vi "iRobot Sensor Stream Process (all sensors).vi"(11 "stream in":u8[](array[numeric])) -> (1 "sensors":T1 {"Infrared" format="%02x"}, 2 "Packet Found?":bool, 3 "stream out":u8[](array[numeric]))   [LabVIEW 2010]
doc: "Process a stream of UART communication and extract a sensor packet.\n\nFor simplicity, this VI assumes that the robot is streaming Sensor Group 6, which contains all sensor data."
uses:
  Sensor Controls/iRobot Sensor Group 6.ctl
  Sensor Controls/iRobot Bumps + Wheel Drops.ctl
  Sensor Controls/iRobot Low-Side Driver + Wheel Overcurrent.ctl
  Sensor Controls/iRobot Buttons.ctl
  Sensor Controls/iRobot Charging State.ctl
  Sensor Controls/iRobot Cargo Bay Digital Inputs.ctl
  Sensor Controls/iRobot Charging Sources Available.ctl
  Sensor Controls/iRobot OI Mode.ctl
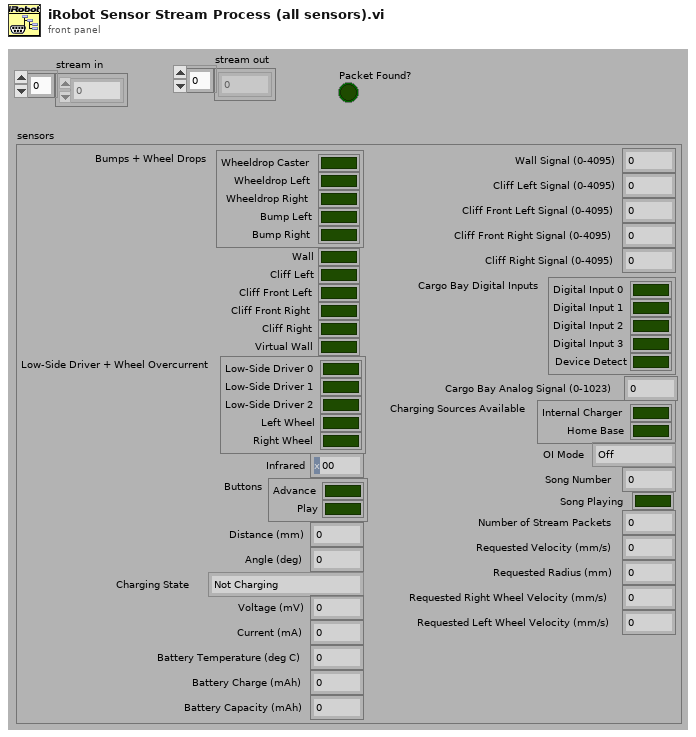
[diagram p1: front panel]
types:
  T1 = typedef "iRobot Sensor Group 6.ctl" = cluster{"Bumps + Wheel Drops":T2, "Wall":bool, "Cliff Left":bool, "Cliff Front Left":bool, "Cliff Front Right":bool, "Cliff Right":bool, "Virtual Wall":bool, "Low-Side Driver + Wheel Overcurrent":T3, "Infrared":u8, "Buttons":T4, "Distance (mm)":i32, "Angle (deg)":i32, "Charging State":T5, "Voltage (mV)":u16, "Current (mA)":i16, "Battery Temperature (deg C)":i8, "Battery Charge (mAh)":u16, "Battery Capacity (mAh)":u16, "Wall Signal (0-4095)":u16, "Cliff Left Signal (0-4095)":u16, "Cliff Front Left Signal (0-4095)":u16, "Cliff Front Right Signal (0-4095)":u16, "Cliff Right Signal (0-4095)":u16, "Cargo Bay Digital Inputs":T6, "Cargo Bay Analog Signal (0-1023)":u16, "Charging Sources Available":T7, "OI Mode":T8, "Song Number":u8, "Song Playing":bool, "Number of Stream Packets":u8, "Requested Velocity (mm/s)":u8, "Requested Radius (mm)":u8, "Requested Right Wheel Velocity (mm/s)":u8, "Requested Left Wheel Velocity (mm/s)":u8}
  T2 = typedef "iRobot Bumps + Wheel Drops.ctl" = cluster{"Wheeldrop Caster":bool, "Wheeldrop Left":bool, "Wheeldrop Right":bool, "Bump Left":bool, "Bump Right":bool}
  T3 = typedef "iRobot Low-Side Driver + Wheel Overcurrent.ctl" = cluster{"Low-Side Driver 0":bool, "Low-Side Driver 1":bool, "Low-Side Driver 2":bool, "Left Wheel":bool, "Right Wheel":bool}
  T4 = typedef "iRobot Buttons.ctl" = cluster{"Advance":bool, "Play":bool}
  T5 = typedef "iRobot Charging State.ctl" = enum16{"Not Charging", "Reconditioning Charging", "Full Charging", "Trickle Charging", "Waiting", "Charging Fault Condition"}
  T6 = typedef "iRobot Cargo Bay Digital Inputs.ctl" = cluster{"Digital Input 0":bool, "Digital Input 1":bool, "Digital Input 2":bool, "Digital Input 3":bool, "Device Detect":bool}
  T7 = typedef "iRobot Charging Sources Available.ctl" = cluster{"Internal Charger":bool, "Home Base":bool}
  T8 = typedef "iRobot OI Mode.ctl" = enum16{"Off", "Passive", "Safe", "Full"}
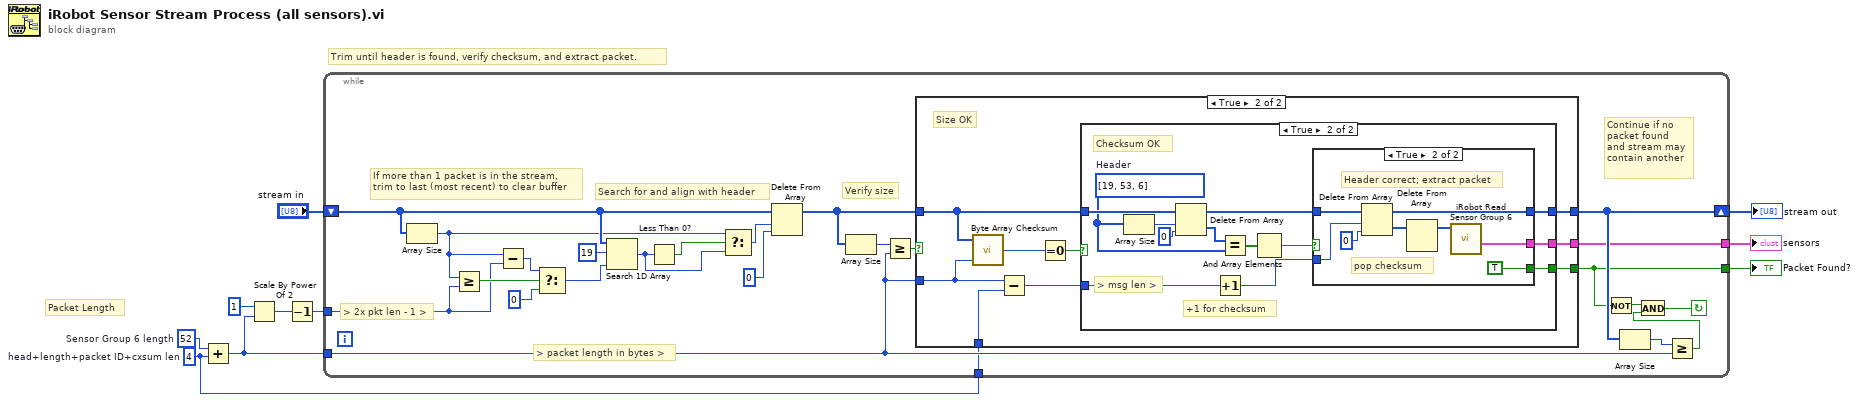
[diagram p0: block diagram]
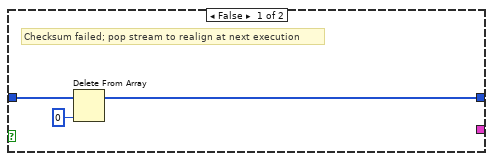
[diagram p3: hidden frame]
diagram:
  w3 = u8 52  # Sensor Group 6 length
  w2 = u8 4  # head+length+packet ID+cxsum len
  # "Packet Length"
  # "Trim until header is found, verify checksum, and extract packet."
  n1 = Add(x=w3, y=w2) -> (x+y=w4:u8)
  n2 = Scale By Power Of 2(n=1, x=w4) -> (x*2^n=w7:u8)
  n3 = Decrement(x=w7) -> (x-1=w5:u8)
  n4 = while {
    shift-right: [w25] -> w9
    shift-left: "stream in" -> [w26]
    tunnel: [w22] -> w8
    tunnel: w5 -> [w18]
    tunnel: w4 -> [w17]
    tunnel: [w14] -> w1
    tunnel: w2 -> [w13]
    stop <- w24 continue-if-true
    # "> 2x pkt len - 1 >"
    # "Continue if no\npacket found\nand stream may\ncontain another"
    # "> packet length in bytes >"
    # "Verify size"
    # "If more than 1 packet is in the stream,\ntrim to last (most recent) to clear buffer"
    # "Search for and align with header"
    n5 = Array Size(array=w26) -> (size(s)=w21:i32)
    n6 = Greater Or Equal?(x=w21, y=w18) -> (x >= y?=w31:bool)
    n7 = Subtract(x=w21, y=w18) -> (x-y=w32:i32)
    n8 = Select(t=w32, s=w31, f=0) -> (s? t:f=w29:i32)
    n9 = Search 1D Array(1D array=w26, element=u8 19 ("y"), start index (0)=w29) -> (index of element=w11:i32)
    n10 = Less Than 0?(x=w11) -> (x < 0?=w12:bool)
    n11 = Select(t=w21, s=w12, f=w11) -> (s? t:f=w20:i32)
    n12 = Delete From Array(array=w26, length=w20, index=0 ("t")) -> (array with subset deleted=w28:u8[])  [unwired: 1 out]
    n13 = Array Size(array=w28) -> (size(s)=w34:i32)
    n14 = Greater Or Equal?(x=w34, y=w17) -> (x >= y?=w27:bool)
    n15 = case shown="True" w27 {
      tunnel: [w35 w44] -> w25
      tunnel: w28 -> [w35 w36]
      tunnel: w17 -> [_ w37]
      tunnel: [_ w41] -> w14
      tunnel: [_ w39] -> w22
      tunnel: w13 -> [_ w38]
      frame False {
        # "Stream is not large enough to contain a full packet"
      }
      frame True {
        # "Size OK"
        n16 = call "Byte Array Checksum.vi"("Number of Values"=w37, "Byte Array"=w36) -> ("Checksum"=w43:u8)  [unwired: 1 in]
        n17 = Subtract(x=w37, y=w38) -> (x-y=w40:u8)
        n18 = Equal To 0?(x=w43) -> (x = 0?=w42:bool)
        n19 = case shown="True" w42 {
          tunnel: w36 -> [w47 w60]
          tunnel: [w46 w57] -> w44
          tunnel: w40 -> [_ w53]
          tunnel: [_ w56] -> w41
          tunnel: [_ w50] -> w39
          frame False {
            # "Checksum failed; pop stream to realign at next execution"
            n20 = Delete From Array(array=w47, index=0) -> (array with subset deleted=w46:u8[])  [unwired: 1 in, 1 out]
          }
          frame True {
            w48 = u8[] [19, 53, 6]  # Header
            # "+1 for checksum"
            # "> msg len >"
            # "Checksum OK"
            n21 = Array Size(array=w48) -> (size(s)=w49:i32)
            n22 = Delete From Array(array=w60, length=w49, index=0) -> (deleted portion=w58:u8[], array with subset deleted=w52:u8[])
            n23 = Increment(x=w53) -> (x+1=w55:u8)
            n24 = Equal?(x=w58, y=w48) -> (x = y?=w54:bool[])
            n25 = And Array Elements(Boolean array=w54) -> (logical AND=w51:bool)
            n26 = case shown="True" w51 {
              tunnel: w52 -> [w61 w69]
              tunnel: w55 -> [_ w68]
              tunnel: [w61 w65] -> w57
              tunnel: [_ w62] -> w56
              tunnel: [_ TRUE] -> w50
              frame False {
                # "Header incorrect"
              }
              frame True {
                # "pop checksum"
                # "Header correct; extract packet"
                n27 = Delete From Array(array=w69, length=w68, index=0) -> (deleted portion=w66:u8[], array with subset deleted=w65:u8[])
                n28 = Delete From Array(array=w66) -> (array with subset deleted=w63:u8[])  [unwired: 2 in, 1 out]
                n29 = call "iRobot Read Sensor Group 6.vi"("stream in"=w63) -> ("iRobot Sensor Group 6"=w62:T1)  [unwired: 9 in, 1 out]
              }
            }
          }
        }
      }
    }
    n30 = Not(x=w22) -> (.not. x?=w15:bool)
    n31 = Array Size(array=w25) -> (size(s)=w23:i32)
    n32 = Greater Or Equal?(x=w23, y=w17) -> (x >= y?=w16:bool)
    n33 = And(x=w15, y=w16) -> (x .and. y?=w24:bool)
  }
  "stream out" <- w9
  "Packet Found?" <- w8
  "sensors" <- w1
